vi "SetAutoscale(SubVI).vi"(8 "error in (no error)":errorcluster, 9 "XYGraph Refnum":refnum<vi>, 10 "Str Refnum":refnum<vi>, 11 "Enum in":refnum<vi>) -> (0 "error out":errorcluster)   [LabVIEW 2018]
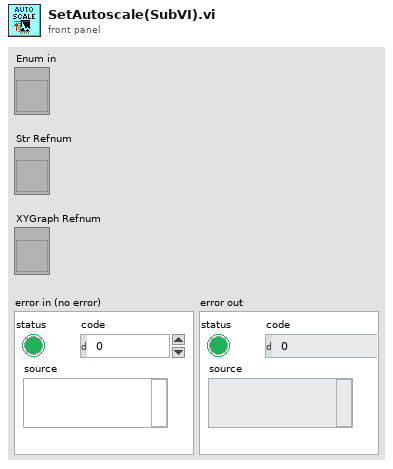
[diagram p1: front panel]
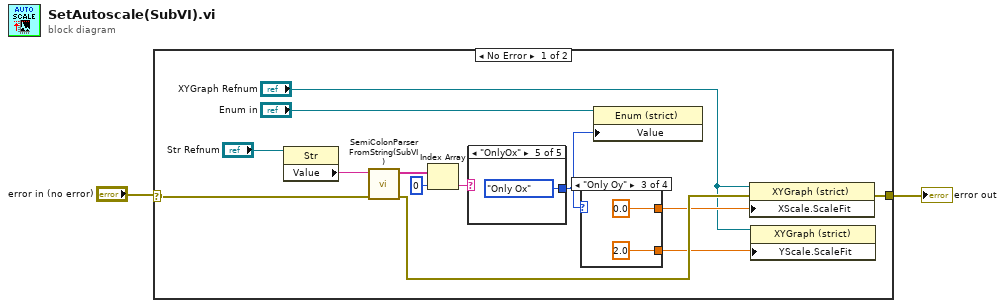
[diagram p0: block diagram]
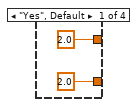
[diagram p2: hidden frame]
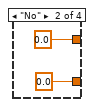
[diagram p3: hidden frame]
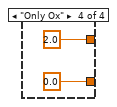
[diagram p4: hidden frame]
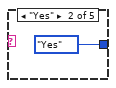
[diagram p6: hidden frame]
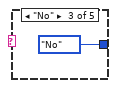
[diagram p7: hidden frame]
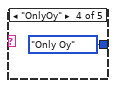
[diagram p8: hidden frame]
diagram:
  n1 = case shown="No Error" "error in (no error)" {
    selector: "error in (no error)" -> [w3 w28]
    tunnel: [w14 w28] -> w2
    frame No Error {
      n2 = property on="Property Node" class="Str"(reference="Str Refnum") -> ("Value"=w8:string)  [unwired: 1 in, 2 out]
      n3 = call "SemiColonParserFromString(SubVI).vi"("Error In"=w3, "String In"=w8) -> ("Error Out"=w15:errorcluster, "String Array Out"=w9:string[])  [unwired: 8 in]
      n4 = Index Array(array=w9, index=0) -> (element=w7:string)
      n5 = case shown="\"OnlyOx\"" w7 {
        tunnel: [_ enum16{"Yes", "No", "Only Oy", "Only Ox"}."Yes" ("Value") enum16{"Yes", "No", "Only Oy", "Only Ox"}."No" ("Value") enum16{"Yes", "No", "Only Oy", "Only Ox"}."Only Oy" ("Value") enum16{"Yes", "No", "Only Oy", "Only Ox"}."Only Ox" ("Value")] -> w10
        frame "False", Default {
        }
        frame "Yes" {
        }
        frame "No" {
        }
        frame "OnlyOy" {
        }
        frame "OnlyOx" {
        }
      }
      n6 = case shown="\"Only Oy\"" w10 {
        tunnel: [2.0 0.0 2.0 0.0] -> w11
        tunnel: [2.0 0.0 0.0 2.0] -> w12
        frame "Yes", Default {
        }
        frame "No" {
        }
        frame "Only Oy" {
        }
        frame "Only Ox" {
        }
      }
      n7 = property on="Property Node" class="Enum (strict)"(reference="Enum in", "Value"=w10) -> ()  [unwired: 1 in, 2 out]
      n8 = property on="Property Node" class="XYGraph (strict)"(reference="XYGraph Refnum", error in=w15, "XScale.ScaleFit"=w12) -> (error out=w14:errorcluster)  [unwired: 1 out]
      n9 = property on="Property Node" class="XYGraph (strict)"(reference="XYGraph Refnum", "YScale.ScaleFit"=w11) -> ()  [unwired: 1 in, 2 out]
    }
    frame Error {
    }
  }
  "error out" <- w2
